vi "XboxGetCommands.vi"(5 "device index":i32) -> (0 "Raw Y":i32, 1 "Raw X":i32, 2 "Prop Command":i32, 3 "Rudder Command":i32)   [LabVIEW 2011]
uses:
  <vilib>/Utility/inputDevices.llb/joystickAcquire.vi
panel:
  out "joysticks info":T1(array[cluster])
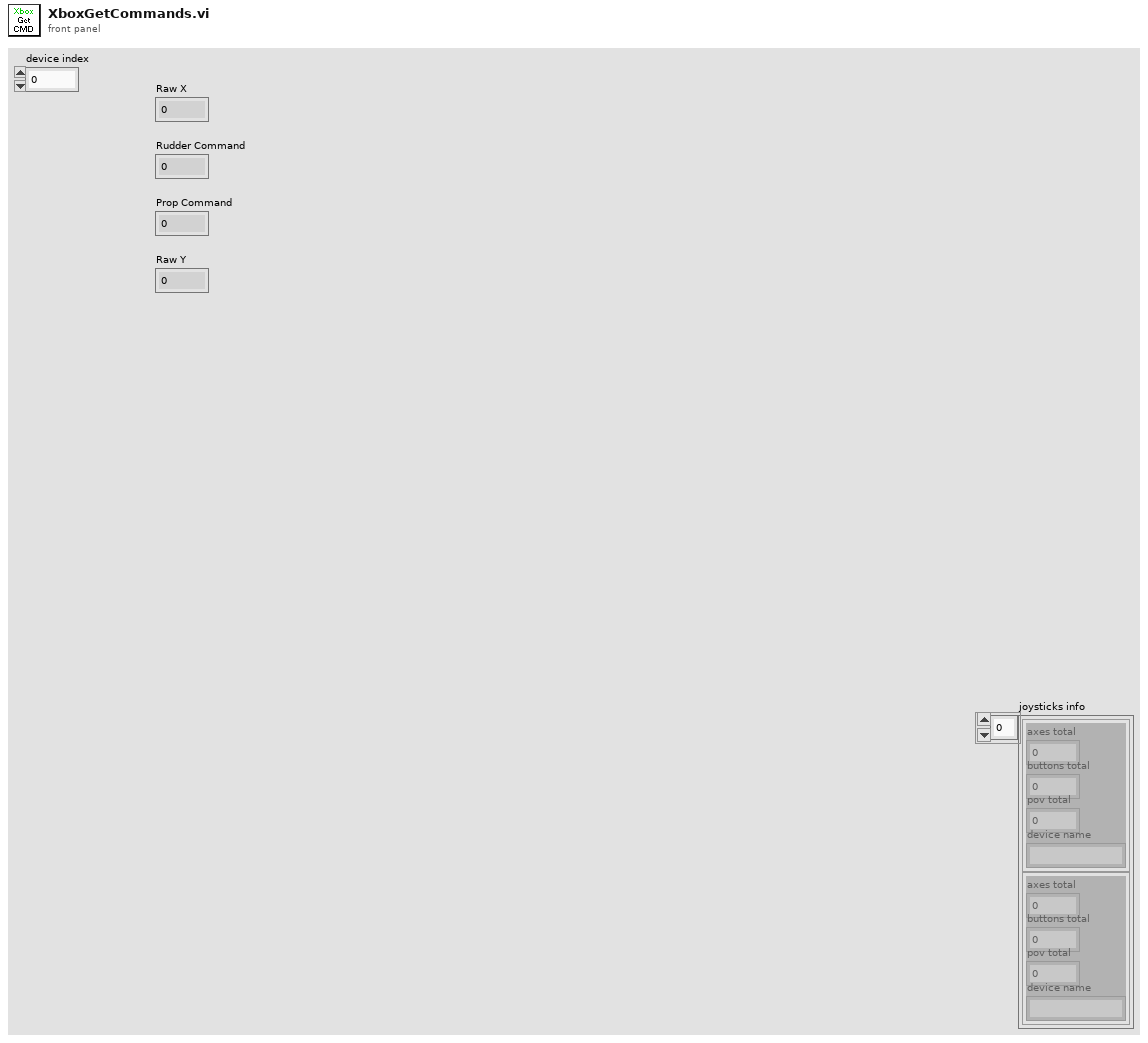
[diagram p1: front panel]
types:
  T1 = cluster{"axes total":u32, "buttons total":u32, "pov total":u32, "device name":string}[]
  T2 = cluster{"X axis":i32, "Y axis":i32, "Z axis":i32, "X axis rotation":i32, "Y axis rotation":i32, "Z axis rotation":i32, "U axis":i32, "V axis":i32}
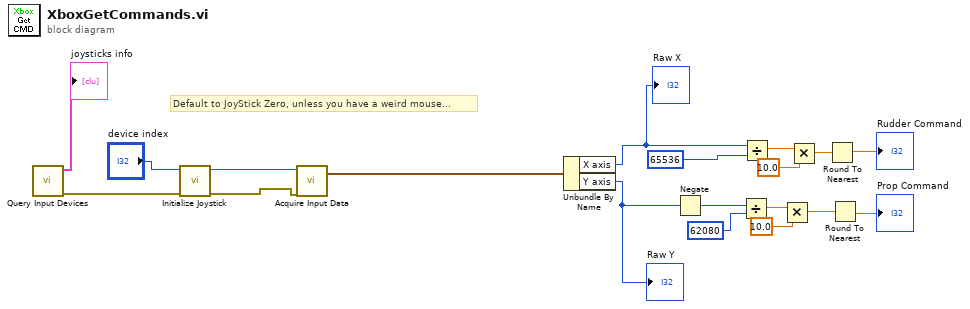
[diagram p0: block diagram]
diagram:
  # "Default to JoyStick Zero, unless you have a weird mouse..."
  n1 = call <vilib>:"Query Input Devices.vi"() -> ("error out"=w6:errorcluster, "joystick info"=→"joysticks info":T1)  [unwired: 1 in, 9 out]
  n2 = call <vilib>:"Initialize Joystick.vi"("error in (no error)"=w6, "device index"="device index") -> ("error out"=w5:errorcluster, "device ID"=w4:refnum<k1>)  [unwired: 8 out]
  n3 = call-poly <vilib>:"Acquire Input Data.vi"("device ID"=w4, "error in (no error)"=w5) -> ("axis info"=w3:T2)  [unwired: 17 out]
  n4 = Unbundle By Name(w3) -> ("X axis"=w11:i32, "Y axis"=w10:i32)
  "Raw X" <- w11
  "Raw Y" <- w10
  n5 = Negate(x=w10) -> (-x=w8:i32)
  n6 = Divide(x=w8, y=62080) -> (x/y=w12:dbl)
  n7 = Divide(x=w11, y=65536) -> (x/y=w15:dbl)
  n8 = Multiply(x=w12, y=10.0) -> (x*y=w17:dbl)
  n9 = Multiply(x=w15, y=10.0) -> (x*y=w16:dbl)
  n10 = Round To Nearest(number=w16) -> (nearest integer value=→"Rudder Command":dbl)
  n11 = Round To Nearest(number=w17) -> (nearest integer value=→"Prop Command":dbl)
